vi "imageParameters.vi"(9 "errorIn":errorcluster, 10 "sessionIn":T2 caption="Session In", 11 "imageIn":T1 caption="Image In") -> (0 "imageHalfRows":i32, 1 "imageHalfCols":i32, 4 "imageCols":i32 caption="Columns", 5 "imageRows":i32 caption="Rows", 6 "errorImageGrab":errorcluster)   [LabVIEW 2021]
uses:
  <vilib>/userdefined/High Color/IMAQdx.ctl
  <vilib>/vision/Image Controls.llb/IMAQ Image.ctl
  <vilib>/vision/driver/NI_Vision_Acquisition_Software.lvlib
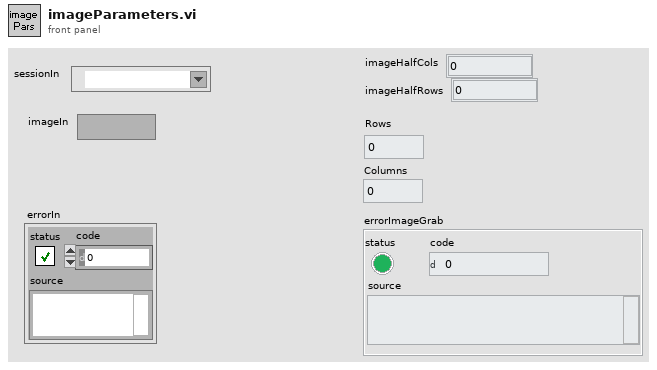
[diagram p1: front panel]
types:
  T1 = typedef "IMAQ Image.ctl" = refnum<image>
  T2 = typedef "IMAQdx.ctl" = refnum<k21>
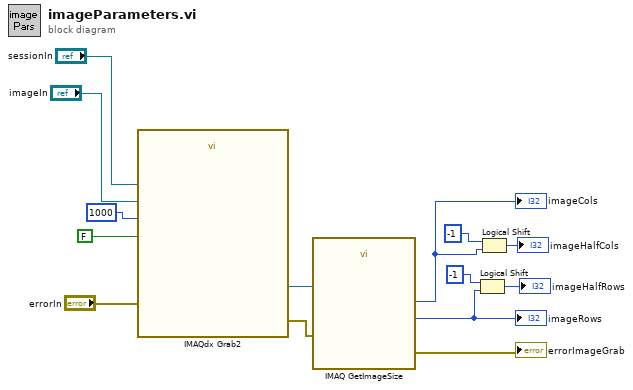
[diagram p0: block diagram]
diagram:
  n1 = call <vilib>:"IMAQdx Grab2.vi"("Timeout (ms)"=1000, "error in"="errorIn", "Wait for Next Buffer? (Yes)"=FALSE, "Image In"="imageIn", "Session In"="sessionIn") -> ("error out"=w5:errorcluster, "Image Out"=w14:T1)  [unwired: 3 in, 2 out]
  n2 = call "IMAQ GetImageSize"("Image"=w14, "error in (no error)"=w5) -> ("Y Resolution"=w7:i32, "X Resolution"=w6:i32, "error out"=→"errorImageGrab":errorcluster)  [unwired: 2 in]
  "imageRows" <- w7
  "imageCols" <- w6
  n3 = Logical Shift(y=-1 ("x"), x=w7) -> (x << y=→"imageHalfRows":i32)
  n4 = Logical Shift(y=-1 ("x"), x=w6) -> (x << y=→"imageHalfCols":i32)
